vi "FTW-Test-Reflection-Array.vi"() -> (0 "Test Result":errorcluster)   [LabVIEW 2015]
uses:
  src/reflection/FTW-Reflection-Types.ctl
  src/core/type/FTW-Type-Actor-Connector.ctl
  src/core/type/FTW-Type-Actor-Inbox.ctl
  src/core/type/FTW-Type-Socket-Publisher.ctl
  src/core/type/FTW-Type-Socket-Subscriber.ctl
  src/core/type/FTW-Type-Socket-Producer.ctl
  src/core/type/FTW-Type-Socket-Consumer.ctl
  src/core/type/FTW-Type-JSON.ctl
  src/core/type/FTW-Type-Regex.ctl
  src/core/type/FTW-Type-SQLite.ctl
  src/reflection/FTW-Reflection-FTWObject.vi
  src/error/FTW-ERR-ThrowInfo.vi
  src/error/FTW-ERR-ThrowError.vi
  src/error/FTW-ERR-CallChain.vi
  src/error/FTW-ERR-NoErrorConstant.vi
  src/string/FTW-STR-ReplaceWhitespace.vi
  src/string/FTW-STR-Array-Delimit.vi
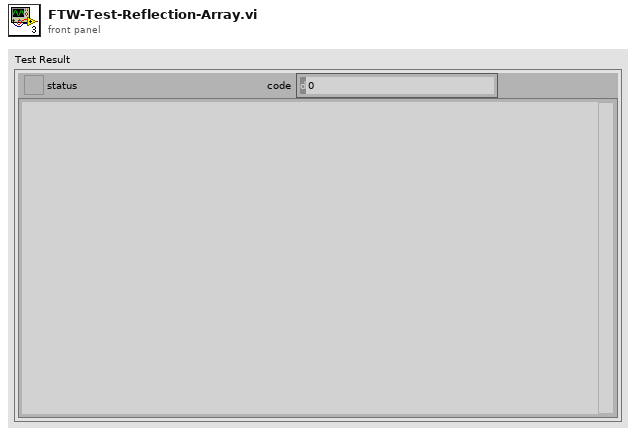
[diagram p1: front panel]
types:
  T1 = typedef "FTW-Reflection-Types.ctl" = enum16{"Unknown", "Void", "Array", "Cluster", "LVObject", "Boolean", "I8", "I16", "I32", "I64", "U8", "U16", "U32", "U64", "SGL", "DBL", "EXT", "CSG", "CDB", "CXT", "FXP", "EnumU8", "EnumU16", "EnumU32", "EnumU64", "SGLwithUnit", "DBLwithUnit", "EXTwithUnit", "CSGwithUnit", "CDBwithUnit", "CXTwithUnit", "String", "Path", "Picture", "Tag", "LVVariant", "Timestamp", "WaveformI8", "WaveformI16", "WaveformI32", "WaveformI64", "WaveformU8", "WaveformU16", "WaveformU32", "WaveformU64", "WaveformSGL", "WaveformDBL", "WaveformEXT", "WaveformCSG", "WaveformCDB", "WaveformCXT", "WaveformDigital", "WaveformUnknownType", "DigitalData", "DynamicData", "ExternalData", "FileByteStream", "TDMStream", "dotNET", "ActiveX", "VIServerReference", "VIReference", "ApplicationInstance", "Menu", "ConnectionDataSocket", "ConnectionVISA", "ConnectionBluetooth", "ConnectionIrDA", "ConnectionTCP", "ConnectionUDP", "ConnectionHTTPClient", "ConnectionFTP", "Occurrence", "Notifier", "Queue", "Rendezvous", "Semaphore", "RTFIFO", "EventPublisher", "EventRegistration", "EventCallback", "DataValueReference", "GenericClass", "GenericClassTag", "GenericClassDeepCopy", "GenericClassFlattened", "GenericClassTagFlattened", "GenericReferenceType", "WindowsRegistry", "OverloadedDatalogRef", "ReferenceUnknownType", "ByteArray", "ConPaneInterface", "FTWObject"}
  T2 = typedef "FTW-Type-Actor-Connector.ctl" = refnum<data-value>
  T3 = typedef "FTW-Type-Actor-Inbox.ctl" = refnum<data-value>
  T4 = typedef "FTW-Type-Socket-Publisher.ctl" = refnum<data-value>
  T5 = typedef "FTW-Type-Socket-Subscriber.ctl" = refnum<data-value>
  T6 = typedef "FTW-Type-Socket-Producer.ctl" = refnum<data-value>
  T7 = typedef "FTW-Type-Socket-Consumer.ctl" = refnum<data-value>
  T8 = typedef "FTW-Type-JSON.ctl" = refnum<data-value>
  T9 = typedef "FTW-Type-Regex.ctl" = refnum<data-value>
  T10 = typedef "FTW-Type-SQLite.ctl" = refnum<data-value>
  T11 = cluster{"Boolean":bool, "U8":u8, "U16":u16, "U32":u32, "U64":u64, "I8":i8, "I16":i16, "I32":i32, "I64":i64, "SGL":sgl, "DBL":dbl, "EXT":ext, "CSG":csg, "CDB":cdb, "CXT":cxt, "FXP":fxp<+/-,64,1024>, "SGLwithUnit":sgl[unit], "DBLwithUnit":dbl[unit], "EXTwithUnit":ext[unit], "CSGwithUnit":csg[unit], "CDBwithUnit":cdb[unit], "CXTwithUnit":cxt[unit], "WaveformU8":waveform(u8), "WaveformU16":waveform(u16), "WaveformU32":waveform(u32), "WaveformU64":waveform(u64), "WaveformI8":waveform(i8), "WaveformI16":waveform(i16), "WaveformI32":waveform(i32), "WaveformI64":waveform(i64), "WaveformSGL":waveform(sgl), "WaveformDBL":waveform(dbl), "WaveformEXT":waveform(ext), "WaveformCSG":waveform(csg), "WaveformCDB":waveform(cdb), "WaveformCXT":waveform(cxt), "WaveformDigital":digitalwaveform, "DynamicData":dynamicdata, "DigitalData":digitaldata, "EnumU8":enum8{"U8"}, "EnumU16":enum16{"U16"}, "EnumU32":enum32{"U32"}, "EnumU32 (Enum U64 doesn't yet exist!)":enum32{"U64"}, "EnumU16 (FTW-Reflection-Types.ctl)":T1, "Array":i32[], "ByteArray":u8[], "Array 2":cluster{"I32":i32}[], "Cluster":cluster{"I32":i32}, "LVObject":refnum<class>, "FileByteStream":refnum<file>, "GenericClass (DOM XML)":refnum<k20>, "TDMStream":refnum<k34>, "OverloadedDatalogRef (Mouse Input Device)":refnum<k1>, "GenericClass (storage refnum)":refnum<k20>, "dotNET":refnum<k24>, "ActiveX":refnum<k7>, "Menu":refnum<k9>, "Picture":picture, "String":string, "Path":path, "ConnectionVISA":refnum<visa-resource-name>, "GenericClassTag (Shared Variable Reference)":refnum<k21>, "GenericClassTag (Network Stream Endpoint)":refnum<k21>, "Notifier":refnum<notifier>, "Queue":refnum<queue>, "EventPublisher":refnum<user-event>, "DataValueReference":refnum<data-value>, "Occurrence":refnum<k4>, "EventCallback":refnum<k27>, "EventRegistration":refnum<event-registration>, "ConnectionIrDA":refnum<k19>, "ConnectionTCP":refnum<k5>, "ConnectionUDP":refnum<k16>, "ConnectionBluetooth":refnum<k31>, "ConnectionDataSocket":refnum<k13>, "VIReference":refnum<vi>, "ApplicationInstance":refnum<vi>, "VIServerReference (Generic Class)":refnum<vi>, "Timestamp":timestamp, "LVVariant":variant, "FTWObject (FTW Actor Connector)":T2, "FTWObject (FTW Actor Inbox)":T3, "FTWObject (FTW Publisher)":T4, "FTWObject (FTW Subscriber)":T5, "FTWObject (FTW Producer)":T6, "FTWObject (FTW Consumer)":T7, "FTWObject (FTW JSON)":T8, "FTWObject (FTW Regex)":T9, "FTWObject (SQLite Connection)":T10}[][][]
  T12 = cluster{"[0]":variant, "[1]":variant, "[2]":variant, "[3]":variant, "[4]":variant, "[5]":variant, "[6]":variant, "[7]":variant, "[8]":variant, "[9]":variant, "[10]":variant, "[11]":variant, "[12]":variant, "[13]":variant, "[14]":variant, "[15]":variant, "[16]":variant, "[17]":variant, "[18]":variant, "[19]":variant, "[20]":variant, "[21]":variant, "[22]":variant, "[23]":variant, "[24]":variant, "[25]":variant, "[26]":variant, "[27]":variant, "[28]":variant, "[29]":variant, "[30]":variant, "[31]":variant, "[32]":variant, "[33]":variant, "[34]":variant, "[35]":variant, "[36]":variant, "[37]":variant, "[38]":variant, "[39]":variant, "[40]":variant, "[41]":variant, "[42]":variant, "[43]":variant, "[44]":variant, "[45]":variant, "[46]":variant, "[47]":variant, "[48]":variant, "[49]":variant, "[50]":variant, "[51]":variant, "[52]":variant, "[53]":variant, "[54]":variant, "[55]":variant, "[56]":variant, "[57]":variant, "[58]":variant, "[59]":variant, "[60]":variant, "[61]":variant, "[62]":variant, "[63]":variant, "[64]":variant, "[65]":variant, "[66]":variant, "[67]":variant, "[68]":variant, "[69]":variant, "[70]":variant, "[71]":variant, "[72]":variant, "[73]":variant, "[74]":variant, "[75]":variant, "[76]":variant, "[77]":variant, "[78]":variant, "[79]":variant, "[80]":variant, "[81]":variant, "[82]":variant, "[83]":variant, "[84]":variant, "[85]":variant, "[86]":variant}
  T13 = cluster{"Element Name":string, "Element Type":T1, "Element Value":variant}[]
  T14 = cluster{"Data Name":string, "LabVIEW Type":T1, "Variant Type and Value":variant}
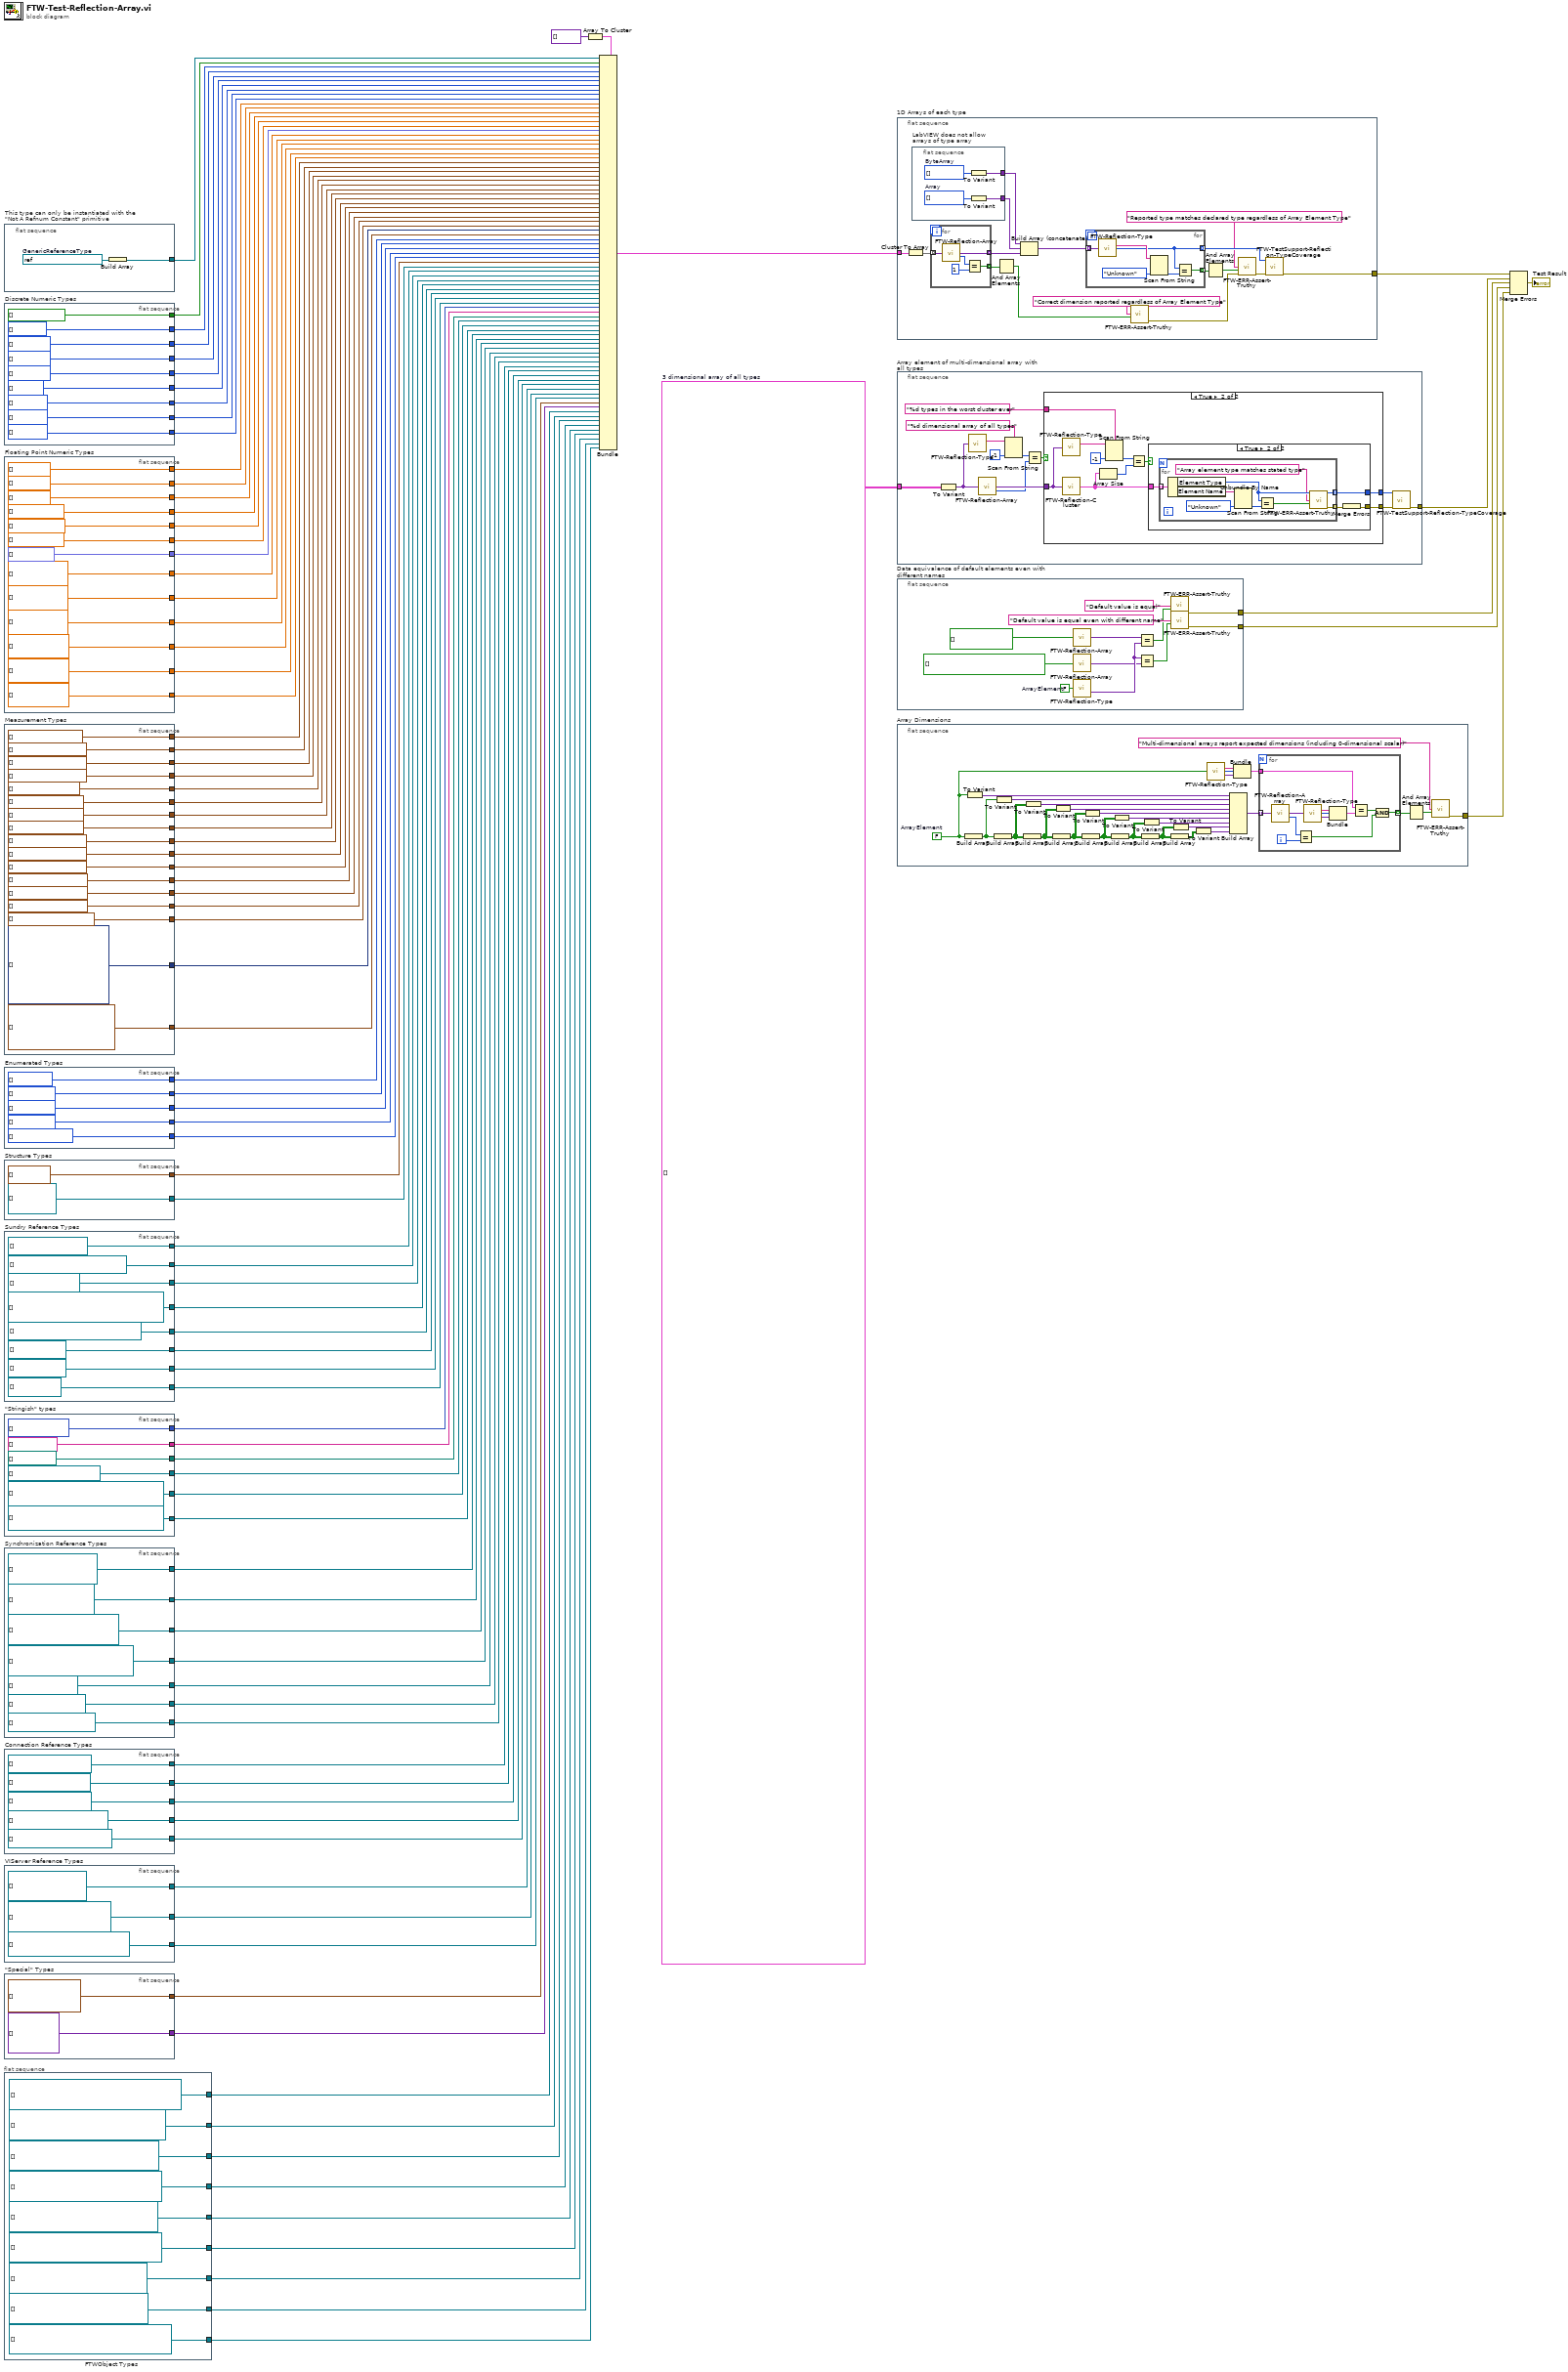
[diagram p0: block diagram]
diagram:
  w97 = T11 []  # 3 dimensional array of all types
  n1 = flat-sequence "This type can only be instantiated with the\n\"Not A Refnum Constant\" primitive" {
    tunnel: [w98] -> w13
    frame #0 {
      w99 = refnum<k0> refnum  # GenericReferenceType
      n2 = Build Array(w99) -> (w98:refnum<k0>[])
    }
  }
  n3 = flat-sequence "Discrete Numeric Types" {
    tunnel: [bool[] []] -> w17
    tunnel: [u8[] []] -> w96
    tunnel: [u16[] []] -> w95
    tunnel: [u32[] []] -> w94
    tunnel: [u64[] []] -> w93
    tunnel: [i8[] []] -> w92
    tunnel: [i16[] []] -> w91
    tunnel: [i32[] []] -> w90
    tunnel: [i64[] []] -> w89
    frame #0 {
    }
  }
  n4 = flat-sequence "Floating Point Numeric Types" {
    tunnel: [sgl[] []] -> w88
    tunnel: [dbl[] []] -> w87
    tunnel: [ext[] []] -> w86
    tunnel: [csg[] []] -> w85
    tunnel: [cdb[] []] -> w84
    tunnel: [cxt[] []] -> w83
    tunnel: [fxp<+/-,64,1024>[] []] -> w82
    tunnel: [sgl[unit][] []] -> w81
    tunnel: [dbl[unit][] []] -> w80
    tunnel: [ext[unit][] []] -> w79
    tunnel: [csg[unit][] []] -> w78
    tunnel: [cdb[unit][] []] -> w77
    tunnel: [cxt[unit][] []] -> w76
    frame #0 {
    }
  }
  n5 = flat-sequence "Measurement Types" {
    tunnel: [waveform(u8)[] []] -> w75
    tunnel: [waveform(u16)[] []] -> w74
    tunnel: [waveform(u32)[] []] -> w73
    tunnel: [waveform(u64)[] []] -> w72
    tunnel: [waveform(i8)[] []] -> w71
    tunnel: [waveform(i16)[] []] -> w70
    tunnel: [waveform(i32)[] []] -> w69
    tunnel: [waveform(i64)[] []] -> w68
    tunnel: [waveform(sgl)[] []] -> w67
    tunnel: [waveform(dbl)[] []] -> w66
    tunnel: [waveform(ext)[] []] -> w65
    tunnel: [waveform(csg)[] []] -> w64
    tunnel: [waveform(cdb)[] []] -> w63
    tunnel: [waveform(cxt)[] []] -> w62
    tunnel: [digitalwaveform[] []] -> w61
    tunnel: [dynamicdata[] []] -> w60
    tunnel: [digitaldata[] []] -> w59
    frame #0 {
    }
  }
  n6 = flat-sequence "Enumerated Types" {
    tunnel: [w143] -> w58
    tunnel: [w142] -> w57
    tunnel: [w141] -> w56
    tunnel: [w140] -> w55
    tunnel: [w139] -> w54
    frame #0 {
      w140 = enum32{"U64"}[] [] items=["U64"]
      w141 = enum32{"U32"}[] [] items=["U32"]
      w142 = enum16{"U16"}[] [] items=["U16"]
      w143 = enum8{"U8"}[] [] items=["U8"]
      w139 = T1[] [] items=["Unknown", "Void", "Array", "Cluster", "LVObject", "Boolean", "I8", "I16", "I32", "I64", "U8", "U16", "U32", "U64", "SGL", "DBL", "EXT", "CSG", "CDB", "CXT", "FXP", "EnumU8", "EnumU16", "EnumU32", "EnumU64", "SGLwithUnit", "DBLwithUnit", "EXTwithUnit", "CSGwithUnit", "CDBwithUnit", "CXTwithUnit", "String", "Path", "Picture", "Tag", "LVVariant", "Timestamp", "WaveformI8", "WaveformI16", "WaveformI32", "WaveformI64", "WaveformU8", "WaveformU16", "WaveformU32", "WaveformU64", "WaveformSGL", "WaveformDBL", "WaveformEXT", "WaveformCSG", "WaveformCDB", "WaveformCXT", "WaveformDigital", "WaveformUnknownType", "DigitalData", "DynamicData", "ExternalData", "FileByteStream", "TDMStream", "dotNET", "ActiveX", "VIServerReference", "VIReference", "ApplicationInstance", "Menu", "ConnectionDataSocket", "ConnectionVISA", "ConnectionBluetooth", "ConnectionIrDA", "ConnectionTCP", "ConnectionUDP", "ConnectionHTTPClient", "ConnectionFTP", "Occurrence", "Notifier", "Queue", "Rendezvous", "Semaphore", "RTFIFO", "EventPublisher", "EventRegistration", "EventCallback", "DataValueReference", "GenericClass", "GenericClassTag", "GenericClassDeepCopy", "GenericClassFlattened", "GenericClassTagFlattened", "GenericReferenceType", "WindowsRegistry", "OverloadedDatalogRef", "ReferenceUnknownType", "ByteArray", "ConPaneInterface", "FTWObject"]
    }
  }
  n7 = flat-sequence "Structure Types" {
    tunnel: [cluster{"I32":i32}[] []] -> w53
    tunnel: [refnum<class>[] []] -> w52
    frame #0 {
    }
  }
  n8 = flat-sequence "Sundry Reference Types" {
    tunnel: [refnum<file>[] []] -> w51
    tunnel: [refnum<k20>[] []] -> w50
    tunnel: [refnum<k34>[] []] -> w49
    tunnel: [w150] -> w48
    tunnel: [refnum<k20>[] []] -> w47
    tunnel: [refnum<k24>[] []] -> w46
    tunnel: [refnum<k7>[] []] -> w45
    tunnel: [refnum<k9>[] []] -> w44
    frame #0 {
      w150 = refnum<k1>[] [] items=["MOUSE"]
    }
  }
  n9 = flat-sequence "\"Stringish\" types" {
    tunnel: [picture[] []] -> w43
    tunnel: [string[] []] -> w42
    tunnel: [path[] []] -> w41
    tunnel: [refnum<visa-resource-name>[] []] -> w40
    tunnel: [refnum<k21>[] []] -> w39
    tunnel: [refnum<k21>[] []] -> w38
    frame #0 {
    }
  }
  n10 = flat-sequence "Synchronization Reference Types" {
    tunnel: [refnum<notifier>[] []] -> w37
    tunnel: [refnum<queue>[] []] -> w36
    tunnel: [refnum<user-event>[] []] -> w35
    tunnel: [refnum<data-value>[] []] -> w34
    tunnel: [refnum<k4>[] []] -> w33
    tunnel: [refnum<k27>[] []] -> w32
    tunnel: [refnum<event-registration>[] []] -> w31
    frame #0 {
    }
  }
  n11 = flat-sequence "Connection Reference Types" {
    tunnel: [refnum<k19>[] []] -> w30
    tunnel: [refnum<k5>[] []] -> w29
    tunnel: [refnum<k16>[] []] -> w28
    tunnel: [refnum<k31>[] []] -> w27
    tunnel: [refnum<k13>[] []] -> w26
    frame #0 {
    }
  }
  n12 = flat-sequence "VIServer Reference Types" {
    tunnel: [refnum<vi>[] []] -> w25
    tunnel: [refnum<vi>[] []] -> w24
    tunnel: [refnum<vi>[] []] -> w23
    frame #0 {
    }
  }
  n13 = flat-sequence "\"Special\" Types" {
    tunnel: [timestamp[] []] -> w22
    tunnel: [variant[] []] -> w21
    frame #0 {
    }
  }
  n14 = flat-sequence "FTWObject Types" {
    tunnel: [T2[] []] -> w9
    tunnel: [T3[] []] -> w8
    tunnel: [T4[] []] -> w7
    tunnel: [T5[] []] -> w6
    tunnel: [T6[] []] -> w5
    tunnel: [T7[] []] -> w4
    tunnel: [T8[] []] -> w3
    tunnel: [T9[] []] -> w2
    tunnel: [T10[] []] -> w1
    frame #0 {
    }
  }
  n15 = Array To Cluster(array=variant[] []) -> (cluster=w15:T12)
  n16 = Bundle(cluster=w15, "[0]"=w13, "[1]"=w17, "[2]"=w96, "[3]"=w95, "[4]"=w94, "[5]"=w93, "[6]"=w92, "[7]"=w91, "[8]"=w90, "[9]"=w89, "[10]"=w88, "[11]"=w87, "[12]"=w86, "[13]"=w85, "[14]"=w84, "[15]"=w83, "[16]"=w82, "[17]"=w81, "[18]"=w80, "[19]"=w79, "[20]"=w78, "[21]"=w77, "[22]"=w76, "[23]"=w75, "[24]"=w74, "[25]"=w73, "[26]"=w72, "[27]"=w71, "[28]"=w70, "[29]"=w69, "[30]"=w68, "[31]"=w67, "[32]"=w66, "[33]"=w65, "[34]"=w64, "[35]"=w63, "[36]"=w62, "[37]"=w61, "[38]"=w60, "[39]"=w59, "[40]"=w58, "[41]"=w57, "[42]"=w56, "[43]"=w55, "[44]"=w54, "[45]"=w53, "[46]"=w52, "[47]"=w51, "[48]"=w50, "[49]"=w49, "[50]"=w48, "[51]"=w47, "[52]"=w46, "[53]"=w45, "[54]"=w44, "[55]"=w43, "[56]"=w42, "[57]"=w41, "[58]"=w40, "[59]"=w39, "[60]"=w38, "[61]"=w37, "[62]"=w36, "[63]"=w35, "[64]"=w34, "[65]"=w33, "[66]"=w32, "[67]"=w31, "[68]"=w30, "[69]"=w29, "[70]"=w28, "[71]"=w27, "[72]"=w26, "[73]"=w25, "[74]"=w24, "[75]"=w23, "[76]"=w22, "[77]"=w21, "[78]"=w9, "[79]"=w8, "[80]"=w7, "[81]"=w6, "[82]"=w5, "[83]"=w4, "[84]"=w3, "[85]"=w2, "[86]"=w1) -> (w14:T12)
  n17 = flat-sequence "1D Arrays of each type" {
    tunnel: [w201] -> w18
    tunnel: w14 -> [w199]
    frame #0 {
      n18 = Cluster To Array(cluster=w199) -> (array=w198:variant[])
      n19 = flat-sequence "LabVIEW does not allow\narrays of type array" {
        tunnel: [w203] -> w196
        tunnel: [w202] -> w195
        frame #0 {
          w204 = i32[] []  # Array
          w205 = u8[] []  # ByteArray
          n20 = To Variant(anything=w205) -> (Variant=w202:variant)
          n21 = To Variant(anything=w204) -> (Variant=w203:variant)
        }
      }
      n22 = for {
        tunnel: [w213] -> w200 mode=indexing
        tunnel: [w212] -> w197 mode=indexing
        tunnel: w198 -> [w214] mode=indexing
        n23 = call "FTW-Reflection-Array.vi"("Array"=w214) -> ("Default Array Element"=w212:variant, "Number of Dimensions"=w216:i32)  [unwired: 13 in]
        n24 = Equal?(x=w216, y=1) -> (x = y?=w213:bool)
      }
      n25 = And Array Elements(Boolean array=w200) -> (logical AND=w189:bool)
      n26 = Build Array (concatenate)(w195, w196, w197) -> (w194:variant[])
      n27 = for {
        tunnel: [w208] -> w190 mode=indexing
        tunnel: w194 -> [w207] mode=indexing
        tunnel: [w206] -> w193 mode=indexing
        n28 = call "FTW-Reflection-Type.vi"("Anything"=w207) -> ("Data Name"=w210:string, "LabVIEW Type"=w208:T1)  [unwired: 12 in, 1 out]
        n29 = Scan From String(input string=w210, default 1=FTW-Reflection-Types."Unknown" ("Element Type")) -> (output 1=w209:T1)  [unwired: 3 in, 3 out]
        n30 = Equal?(x=w208, y=w209) -> (x = y?=w206:bool)
      }
      n31 = call "FTW-ERR-Assert-Truthy.vi"("Assertion"="Correct dimension reported regardless of Array Element Type", "Assertion holds true?"=w189) -> ("error out"=w192:errorcluster)  [unwired: 13 in]
      n32 = And Array Elements(Boolean array=w193) -> (logical AND=w187:bool)
      n33 = call "FTW-ERR-Assert-Truthy.vi"("Assertion"="Reported type matches declared type regardless of Array Element Type", "Assertion holds true?"=w187, "error in"=w192) -> ("error out"=w191:errorcluster)  [unwired: 12 in]
      n34 = call "FTW-TestSupport-Reflection-TypeCoverage.vi"("Types Tested"=w190, "error in"=w191) -> ("error out"=w201:errorcluster)  [unwired: 13 in]
    }
  }
  n35 = flat-sequence "Array element of multi-dimensional array with all types" {
    tunnel: w97 -> [w229]
    tunnel: [w219] -> w20
    frame #0 {
      n36 = To Variant(anything=w229) -> (Variant=w227:variant)
      n37 = call "FTW-Reflection-Type.vi"("Anything"=w227) -> ("Data Name"=w226:string)  [unwired: 12 in, 2 out]
      n38 = call "FTW-Reflection-Array.vi"("Array"=w227) -> ("Default Array Element"=w228:variant, "Number of Dimensions"=w222:i32)  [unwired: 13 in]
      n39 = Scan From String(format string="%d dimensional array of all types", input string=w226, default 1=-1 ("default value 1")) -> (output 1=w221:i32)  [unwired: 2 in, 3 out]
      n40 = Equal?(x=w221, y=w222) -> (x = y?=w220:bool)
      n41 = case shown="True" w220 {
        tunnel: [_ w239] -> w218
        tunnel: w228 -> [_ w232]
        tunnel: "%d types in the worst cluster ever" ("format string") -> [_ w231]
        tunnel: [_ w230] -> w217
        frame False {
        }
        frame True {
          n42 = call "FTW-Reflection-Type.vi"("Anything"=w232) -> ("Data Name"=w238:string)  [unwired: 12 in, 2 out]
          n43 = call "FTW-Reflection-Cluster.vi"("Cluster"=w232) -> ("Cluster Elements"=w236:T13)  [unwired: 14 in]
          n44 = Array Size(array=w236) -> (size(s)=w234:i32)
          n45 = Scan From String(format string=w231, input string=w238, default 1=-1 ("default value 1")) -> (output 1=w235:i32)  [unwired: 2 in, 3 out]
          n46 = Equal?(x=w235, y=w234) -> (x = y?=w233:bool)
          n47 = case shown="True" w233 {
            tunnel: w236 -> [_ w243]
            tunnel: [_ w242] -> w239
            tunnel: [_ w240] -> w230
            frame False {
            }
            frame True {
              n48 = for {
                tunnel: w243 -> [w251] mode=indexing
                tunnel: [w247] -> w242 mode=indexing
                tunnel: [w244] -> w241 mode=indexing
                n49 = Unbundle By Name(w251) -> ("Element Type"=w247:T1, "Element Name"=w248:string)
                n50 = Scan From String(input string=w248, default 1=FTW-Reflection-Types."Unknown" ("Element Type")) -> (output 1=w249:T1)  [unwired: 3 in, 3 out]
                n51 = Equal?(x=w247, y=w249) -> (x = y?=w246:bool)
                n52 = call "FTW-ERR-Assert-Truthy.vi"("Assertion"="Array element type matches stated type", "Assertion holds true?"=w246) -> ("error out"=w244:errorcluster)  [unwired: 13 in]
              }
              n53 = Merge Errors(w241) -> (w240:errorcluster)
            }
          }
        }
      }
      n54 = call "FTW-TestSupport-Reflection-TypeCoverage.vi"("Types Tested"=w218, "error in"=w217) -> ("error out"=w219:errorcluster)  [unwired: 13 in]
    }
  }
  n55 = flat-sequence "Data equivalence of default elements even with different names" {
    tunnel: [w253] -> w11
    tunnel: [w252] -> w10
    frame #0 {
      w261 = FALSE  # ArrayElement
      n56 = call "FTW-Reflection-Array.vi"("Array"=bool[] []) -> ("Default Array Element"=w260:variant)  [unwired: 13 in, 1 out]
      n57 = call "FTW-Reflection-Array.vi"("Array"=bool[] []) -> ("Default Array Element"=w258:variant)  [unwired: 13 in, 1 out]
      n58 = call "FTW-Reflection-Type.vi"("Anything"=w261) -> ("Variant Type and Value"=w259:variant)  [unwired: 12 in, 2 out]
      n59 = Equal?(x=w260, y=w259) -> (x = y?=w254:bool)
      n60 = Equal?(x=w259, y=w258) -> (x = y?=w257:bool)
      n61 = call "FTW-ERR-Assert-Truthy.vi"("Assertion"="Default value is equal", "Assertion holds true?"=w254) -> ("error out"=w253:errorcluster)  [unwired: 13 in]
      n62 = call "FTW-ERR-Assert-Truthy.vi"("Assertion"="Default value is equal even with different name", "Assertion holds true?"=w257) -> ("error out"=w252:errorcluster)  [unwired: 13 in]
    }
  }
  n63 = flat-sequence "Array Dimensions" {
    tunnel: [w272] -> w12
    frame #0 {
      w264 = FALSE  # ArrayElement
      n64 = Build Array(w264) -> (w290:bool[])
      n65 = To Variant(anything=w264) -> (Variant=w265:variant)
      n66 = Build Array(w290) -> (w289:bool[][])
      n67 = To Variant(anything=w290) -> (Variant=w288:variant)
      n68 = Build Array(w289) -> (w284:bool[][][])
      n69 = To Variant(anything=w289) -> (Variant=w285:variant)
      n70 = Build Array(w284) -> (w281:bool[][][][])
      n71 = To Variant(anything=w284) -> (Variant=w283:variant)
      n72 = Build Array(w281) -> (w286:bool[][][][][])
      n73 = To Variant(anything=w281) -> (Variant=w282:variant)
      n74 = Build Array(w286) -> (w287:bool[][][][][][])
      n75 = To Variant(anything=w286) -> (Variant=w280:variant)
      n76 = Build Array(w287) -> (w278:bool[][][][][][][])
      n77 = To Variant(anything=w287) -> (Variant=w279:variant)
      n78 = Build Array(w278) -> (w277:bool[][][][][][][][])
      n79 = To Variant(anything=w278) -> (Variant=w276:variant)
      n80 = To Variant(anything=w277) -> (Variant=w275:variant)
      n81 = call "FTW-Reflection-Type.vi"("Anything"=w264) -> ("Data Name"=w271:string, "LabVIEW Type"=w269:T1, "Variant Type and Value"=w270:variant)  [unwired: 12 in]
      n82 = Build Array(w265, w288, w285, w283, w282, w280, w279, w276, w275) -> (w274:variant[])
      n83 = Bundle("Data Name"=w271, "LabVIEW Type"=w269, "Variant Type and Value"=w270) -> (w268:T14)  [unwired: 1 in]
      n84 = for {
        tunnel: w274 -> [w302] mode=indexing
        tunnel: [w293] -> w273 mode=indexing
        tunnel: w268 -> [w300]
        i -> [w291]
        n85 = call "FTW-Reflection-Array.vi"("Array"=w302) -> ("Default Array Element"=w296:variant, "Number of Dimensions"=w301:i32)  [unwired: 13 in]
        n86 = Equal?(x=w301, y=w291) -> (x = y?=w295:bool)
        n87 = call "FTW-Reflection-Type.vi"("Anything"=w296) -> ("Data Name"=w297:string, "LabVIEW Type"=w299:T1, "Variant Type and Value"=w298:variant)  [unwired: 12 in]
        n88 = Bundle("Data Name"=w297, "LabVIEW Type"=w299, "Variant Type and Value"=w298) -> (w292:T14)  [unwired: 1 in]
        n89 = Equal?(x=w300, y=w292) -> (x = y?=w294:bool)
        n90 = Compound Arithmetic op=AND(w294, w295) -> (w293:bool)
      }
      n91 = And Array Elements(Boolean array=w273) -> (logical AND=w267:bool)
      n92 = call "FTW-ERR-Assert-Truthy.vi"("Assertion"="Multi-dimensional arrays report expected dimensions (including 0-dimensional scalar)", "Assertion holds true?"=w267) -> ("error out"=w272:errorcluster)  [unwired: 13 in]
    }
  }
  n93 = Merge Errors(w18, w20, w11, w10, w12) -> (→"Test Result":errorcluster)
